vi "Read Marker (Reference Marker).vi"(0 "VISA resource name":refnum<visa-resource-name>, 7 "Marker (0:Frequency & Time)":i32(ring) items=["Frequency & Time", "Level", "Position"], 11 "error in (no error)":errorcluster) -> (4 "VISA resource name out":refnum<visa-resource-name>, 6 "Reference Marker Response":dbl format="%.3f", 15 "error out":errorcluster)   [LabVIEW 2023, in "Anritsu Signal Analyzer Series.lvlib"]
doc: "Reads the Reference Marker data."
uses:
  Anritsu Signal Analyzer Series.lvlib
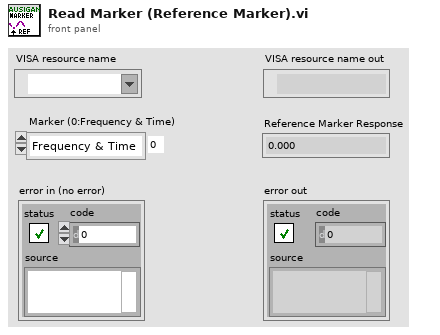
[diagram p1: front panel]
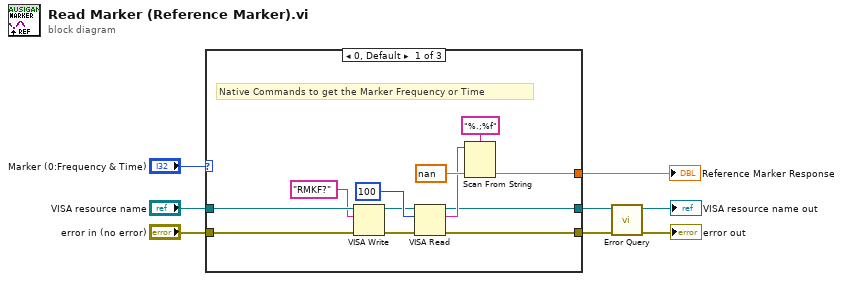
[diagram p0: block diagram]
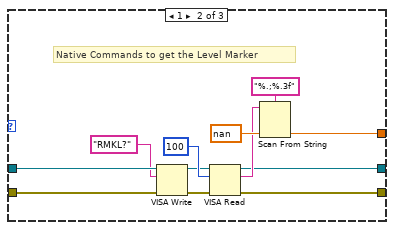
[diagram p2: hidden frame]
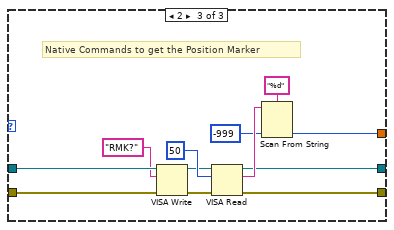
[diagram p3: hidden frame]
diagram:
  n1 = case shown="0, Default" "Marker (0:Frequency & Time)" {
    tunnel: "error in (no error)" -> [w15 w27 w40]
    tunnel: "VISA resource name" -> [w14 w26 w39]
    tunnel: [w13 w25 w38] -> w2
    tunnel: [w12 w24 w37] -> w1
    tunnel: [w11 w23 w36] -> w4
    frame 0, Default {
      # "Native Commands to get the Marker Frequency or Time"
      n2 = VISA Write(VISA resource name=w14, write buffer="RMKF?" ("_Command"), error in (no error)=w15) -> (VISA resource name out=w16:refnum<visa-resource-name>, error out=w17:errorcluster)  [unwired: 1 out]
      n3 = VISA Read(VISA resource name=w16, byte count=u32 100 ("byte count (0)"), error in (no error)=w17) -> (VISA resource name out=w13:refnum<visa-resource-name>, read buffer=w19:string, error out=w12:errorcluster)  [unwired: 1 out]
      n4 = Scan From String(format string="%.;%f" ("Format String"), input string=w19, default 1=nan ("_Default")) -> (output 1=w11:dbl)  [unwired: 2 in, 3 out]
    }
    frame 1 {
      # "Native Commands to get the Level Marker"
      n5 = VISA Write(VISA resource name=w26, write buffer="RMKL?" ("_Command"), error in (no error)=w27) -> (VISA resource name out=w28:refnum<visa-resource-name>, error out=w29:errorcluster)  [unwired: 1 out]
      n6 = VISA Read(VISA resource name=w28, byte count=u32 100 ("byte count (0)"), error in (no error)=w29) -> (VISA resource name out=w25:refnum<visa-resource-name>, read buffer=w31:string, error out=w24:errorcluster)  [unwired: 1 out]
      n7 = Scan From String(format string="%.;%.3f" ("Format String"), input string=w31, default 1=nan ("_Default")) -> (output 1=w23:dbl)  [unwired: 2 in, 3 out]
    }
    frame 2 {
      # "Native Commands to get the Position Marker"
      n8 = VISA Write(VISA resource name=w39, write buffer="RMK?" ("_Command"), error in (no error)=w40) -> (VISA resource name out=w41:refnum<visa-resource-name>, error out=w42:errorcluster)  [unwired: 1 out]
      n9 = VISA Read(VISA resource name=w41, byte count=u32 50 ("byte count (0)"), error in (no error)=w42) -> (VISA resource name out=w38:refnum<visa-resource-name>, read buffer=w44:string, error out=w37:errorcluster)  [unwired: 1 out]
      n10 = Scan From String(format string="%d" ("Format String"), input string=w44, default 1=-999 ("_Default")) -> (output 1=w36:i32)  [unwired: 2 in, 3 out]
    }
  }
  "Reference Marker Response" <- w4
  n11 = call "Error Query.vi"("error in (no error)"=w1, "VISA resource name"=w2) -> ("error out"=→"error out":errorcluster, "VISA resource name out"=→"VISA resource name out":refnum<visa-resource-name>)  [unwired: 6 in, 2 out]
